vi "Write.vi"(5 "Finished? (True)":bool=TRUE, 6 "Mask payload?":bool, 7 "Opcode (Text)":T1=1 items=["Cont. Frame"=0, "Text"=1, "Binary"=2, "Ping"=9, "Pong"=10], 8 "error in (no error)":errorcluster, 9 "timeout ms (5000)":i32=5000, 10 "Data":string, 11 "WebSocket in":refnum<class "WebSocket.lvclass">) -> (0 "error out":errorcluster, 3 "WebSocket out":refnum<class "WebSocket.lvclass">)   [LabVIEW 2021, in "WebSockets.lvlib"]
doc: "**Deprecated - please use the new WebSocket.lvclass VIs instead. VI is retained for backwards compatibility.**\n\nSends a WebSocket message to the client. Messages sent from the client must be masked but it is optional for the server.\n\nFinished should be set to True unless sending a fragmented message.\nWebSockets 2.0.1.40\nSam Sharp - MediaMongrels Ltd\nCopyright (c) 2019, MediaMongrels Ltd"
uses:
  WebSockets.lvlib
  WebSocket/WebSocket.lvclass
  WebSocket/Opcodes.ctl
  WebSocket/WebSocket.lvclass/WebSocket.ctl
  WebSocket/DataLengthBytes.vi
  WebSocket/EncodeMaskedBytes.vi
  Sockets/Socket/Socket.lvclass
panel:
  # "(leave as 'True' unless sending fragmented messages)"
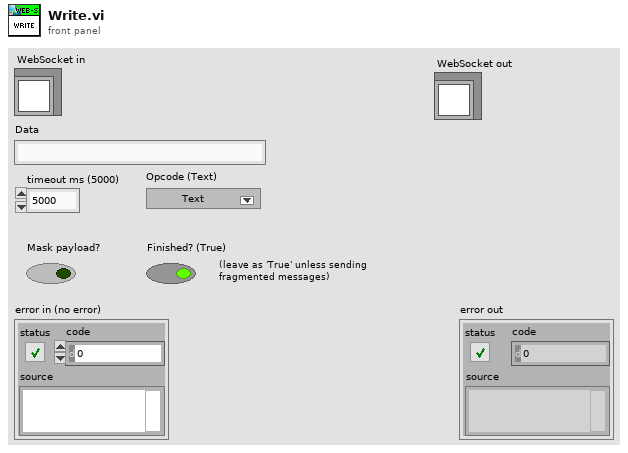
[diagram p1: front panel]
types:
  T1 = typedef "WebSockets.lvlib/WebSocket.lvclass/Opcodes.ctl" = u8
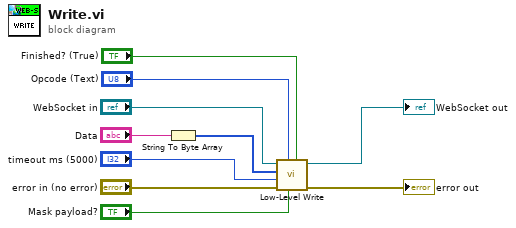
[diagram p0: block diagram]
diagram:
  n1 = String To Byte Array(string="Data") -> (unsigned byte array=w1:u8[])
  n2 = call "Low-Level Write.vi"("Finished? (True)"="Finished? (True)", "Mask payload?"="Mask payload?", "Opcode (Text)"="Opcode (Text)", "error in (no error)"="error in (no error)", "timeout ms (5000)"="timeout ms (5000)", "Data"=w1, "WebSockets in"="WebSocket in") -> ("error out"=→"error out":errorcluster, "WebSockets out"=→"WebSocket out":refnum<class "WebSocket.lvclass">)  [unwired: 2 in, 1 out]
